vi "device ui.vi"(10 "UI VI Ref (empty)":refnum<vi>, 11 "Template in":refnum<class "Template.lvclass">) -> ()   [LabVIEW 2020, in "Template.lvlib" / "Template.lvclass"]
doc: "Overrides the UI method.\nThis is UI is either launched inside the controller's designated space for UI overrides or as a stand alone pop-up window."
uses:
  Template.lvclass
  Template.lvclass/Template.ctl
panel:
  out "i":i32
  in  "stop":bool
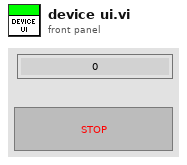
[diagram p1: front panel]
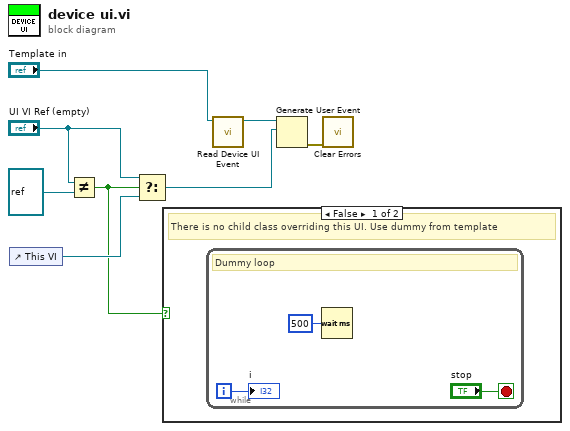
[diagram p0: block diagram]
diagram:
  n1 = control-ref of="This VI"() -> (w4:refnum<vi>)
  n2 = Not Equal?(x="UI VI Ref (empty)", y=refnum<vi> refnum ("This VI")) -> (x != y?=w2:bool)
  n3 = Select(t="UI VI Ref (empty)", s=w2, f=w4) -> (s? t:f=w3:refnum<vi>)
  n4 = case shown="False" w2 {
    frame False {
      # "There is no child class overriding this UI. Use dummy from template"
      n5 = while {
        i -> [w9]
        stop <- "stop" stop-if-true
        # "Dummy loop"
        n6 = Wait (ms)(milliseconds to wait=u32 500) -> ()  [unwired: 1 out]
        "i" <- w9
      }
    }
    frame True {
      # "A child class is overriding this method.\nDon't lock it."
    }
  }
  n7 = call "Read Device UI Event.vi"("Template in"="Template in") -> ("Device UI Event"=w8:refnum<user-event>)  [unwired: 10 in]
  n8 = Generate User Event(user event=w8, event data cluster=w3) -> (error out=w1:errorcluster)  [unwired: 2 in, 1 out]
  n9 = call <vilib>:"Clear Errors.vi"("error in (no error)"=w1) -> ()  [unwired: 5 in, 2 out]
